vi "Close Device Core.vi"(8 "error in (no error)":errorcluster, 11 "CS++IEFWerner in":refnum<class "CS++IEFWerner.lvclass">) -> (0 "error out":errorcluster, 3 "CS++IEFWerner out":refnum<class "CS++IEFWerner.lvclass">)   [LabVIEW 2015, in "CS++IEFWerner.lvlib" / "CS++IEFWerner.lvclass"]
doc: "Close device driver connection."
uses:
  CS++IEFWerner.lvclass
  CSPP_DeviceBase/CS++Motor/CS++Motor.lvclass
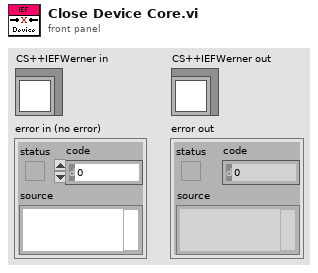
[diagram p1: front panel]
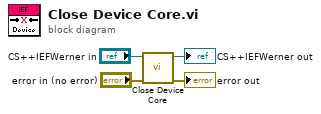
[diagram p0: block diagram]
diagram:
  n1 = call-parent "Close Device Core.vi"("error in (no error)"="error in (no error)", "CS++Motor in"="CS++IEFWerner in") -> ("error out"=→"error out":errorcluster, "CS++Motor out"=→"CS++IEFWerner out":refnum<class "CS++IEFWerner.lvclass">)  [unwired: 8 in]
